vi "PH_OceanOpticsSpectrometer.Initialize Device.vi"(0 "i ref in":refnum<vi>, 5 "error in (no error)":errorcluster) -> (14 "i ref out":refnum<vi>, 19 "error out":errorcluster)   [LabVIEW 2014, in "PH_OceanOpticsSpectrometer.lvlib"]
doc: "This VI reads the spectra out of the device and indicates the data."
uses:
  PH_OceanOpticsSpectrometer.lvlib
  PH_OceanOpticsSpectrometer.Trigger.ctl
  PH_StatusHandler/PH_StatusHandler.lvlib
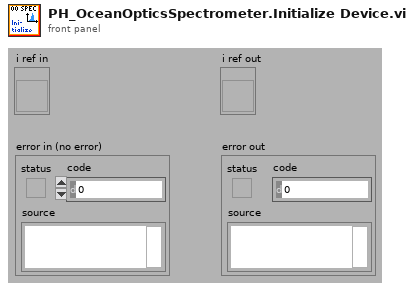
[diagram p1: front panel]
types:
  T1 = typedef "PH_StatusHandler.lvlib/PH_StatusHandler.Status.ctl" = i16
  T2 = typedef "PH_OceanOpticsSpectrometer.lvlib/PH_OceanOpticsSpectrometer.Trigger.ctl" = enum32{"External", "Normal"}
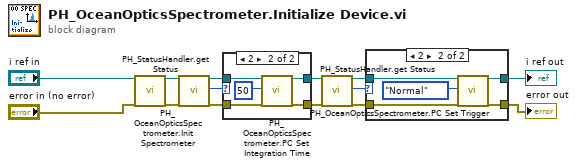
[diagram p0: block diagram]
diagram:
  n1 = call "PH_OceanOpticsSpectrometer.Init Spectrometer.vi"("i ref in"="i ref in", "error in"="error in (no error)") -> ("i ref out"=w8:refnum<vi>, "error out"=w10:errorcluster)  [unwired: 16 in]
  n2 = call "PH_StatusHandler.get Status.vi"("VI in"=w8, "error in"=w10) -> ("VI out"=w7:refnum<vi>, "Status"=w6:T1, "error out"=w9:errorcluster)  [unwired: 15 in]
  n3 = case shown="2" w6 {
    tunnel: [w15 w20] -> w4
    tunnel: [w16 w19] -> w2
    tunnel: w9 -> [w15 w18]
    tunnel: w7 -> [w16 w17]
    frame Default {
    }
    frame 2 {
      n4 = call "PH_OceanOpticsSpectrometer.PC Set Integration Time.vi"("VI in"=w17, "Wanted Integration Time [ms]"=u16 50, "error in (no error)"=w18) -> ("VI out"=w19:refnum<vi>, "error out"=w20:errorcluster)  [unwired: 15 in]
    }
  }
  n5 = call "PH_StatusHandler.get Status.vi"("VI in"=w2, "error in"=w4) -> ("VI out"=w3:refnum<vi>, "Status"=w1:T1, "error out"=w5:errorcluster)  [unwired: 15 in]
  n6 = case shown="2" w1 {
    tunnel: [w22 w28] -> w14
    tunnel: [w23 w26] -> w13
    tunnel: w5 -> [w22 w25]
    tunnel: w3 -> [w23 w24]
    frame Default {
    }
    frame 2 {
      n7 = call "PH_OceanOpticsSpectrometer.PC Set Trigger.vi"("VI in"=w24, "Wanted Trigger"=PH_OceanOpticsSpectrometer.Trigger."Normal", "error in (no error)"=w25) -> ("VI out"=w26:refnum<vi>, "error out"=w28:errorcluster)  [unwired: 15 in]
    }
  }
  "error out" <- w14
  "i ref out" <- w13
